vi "instrumentsInitialization.vi"(8 "error in":errorcluster, 11 "Instrument VISA in":T1={"AWG VISA"="AGTMY51400121", "Oscilloscope  VISA "="labosc4", "Integration Board IP"="172.16.7.43", "connection ID"=refnum, "report out"=refnum, "report file path"=path "C:/CTA/LevelTriggerBoardTest/TestsData/sumtrigger_delay/tmp"}) -> (0 "error out":errorcluster, 3 "Instrument VISA out":T1)   [LabVIEW 2012]
doc: "This VI initializes all the instrumentation needed to carry on several tests and also, establishes the communication with the Integration Board."
uses:
  <vilib>/Utility/NIReport.llb/NI_report.lvclass
  Sum_Abrilader/L0_Sum_Adder Folder/C/Program Files/National Instruments/LabVIEW 2012/instr.lib/Agilent 81150/Agilent 81150.lvlib
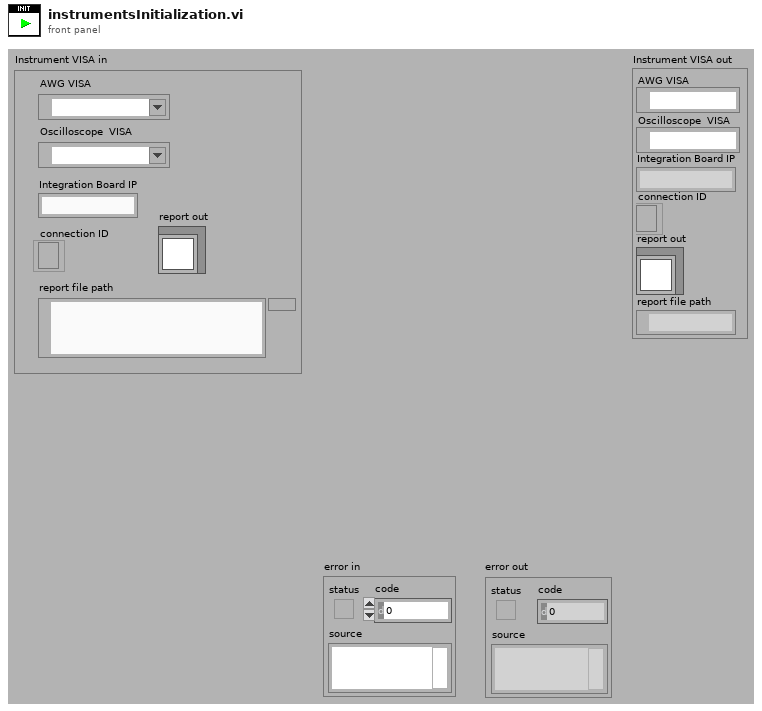
[diagram p1: front panel]
types:
  T1 = cluster{"AWG VISA":refnum<visa-resource-name>, "Oscilloscope  VISA ":refnum<visa-resource-name>, "Integration Board IP":string, "connection ID":refnum<k5>, "report out":refnum<class "NI_report.lvclass">, "report file path":path}
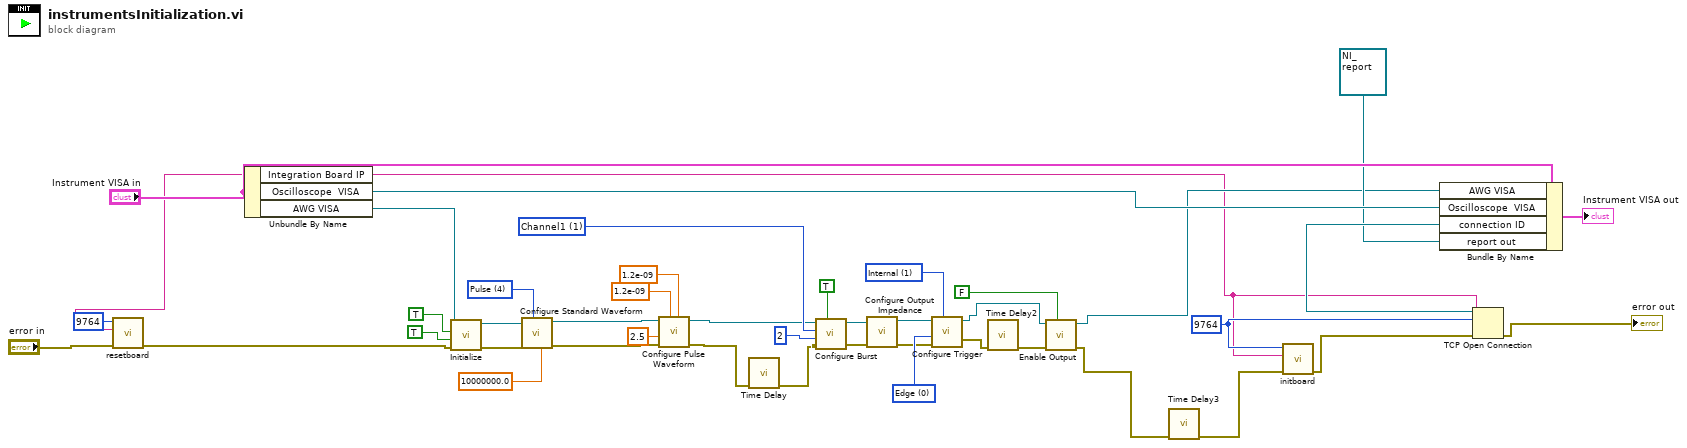
[diagram p0: block diagram]
diagram:
  w27 = u16 1 items=["Channel1"=1, "Channel2"=2] ("Channel (1: Channel1)")
  w34 = u16 4 items=["Sine", "Square", "Ramp Up", "Ramp Down", "Pulse", "Noise", "DC"] ("Waveform (0: Sine)")
  w6 = u16 9764 ("remote port or service name")
  w38 = u16 1 items=["Immediate", "Internal", "External", "Software Trigger Function"] ("Trigger Source (0: Immediate)")
  w43 = u16 0 items=["Edge", "Level"] ("Trigger Mode (0: Edge)")
  n1 = Unbundle By Name("Instrument VISA in") -> ("Integration Board IP"=w5:string, "Oscilloscope  VISA"=w23:refnum<visa-resource-name>, "AWG VISA"=w37:refnum<visa-resource-name>)
  n2 = call "resetboard.vi"("error in (no error)"="error in", "address"=w5, "remote port or service name"=u16 9764) -> ("error out"=w4:errorcluster)  [unwired: 7 in, 1 out]
  n3 = call <instrlib>:"Initialize.vi"("error in (no error)"=w4, "Reset (True)"=TRUE, "ID Query (True)"=TRUE, "VISA resource name"=w37) -> ("error out"=w32:errorcluster, "VISA resource name out"=w33:refnum<visa-resource-name>)  [unwired: 6 in]
  n4 = call <instrlib>:"Configure Standard Waveform.vi"("Frequency (1000.0 Hz)"=10000000.0, "Waveform (0: Sine)"=w34, "error in (no error)"=w32, "VISA resource name"=w33) -> ("error out"=w15:errorcluster, "VISA resource name out"=w13:refnum<visa-resource-name>)  [unwired: 6 in]
  n5 = call <instrlib>:"Configure Pulse Waveform.vi"("Trailing Edge Time (7.5E-9 Seconds)"=1.2e-09, "Leading Edge Time (7.5E-9 Seconds)"=1.2e-09, "error in (no error)"=w15, "Duty Cycle (50.0 %)"=2.5, "VISA resource name"=w13) -> ("error out"=w14:errorcluster, "VISA resource name out"=w12:refnum<visa-resource-name>)  [unwired: 5 in]
  n6 = call "Time Delay"("error in (no error)"=w14) -> ("error out"=w28:errorcluster)  [unwired: 10 in]
  n7 = call <instrlib>:"Configure Burst.vi"("Enable Burst (F: Disable)"=TRUE, "error in (no error)"=w28, "Burst Count (2)"=2, "Channel (1: Channel1)"=w27, "VISA resource name"=w12) -> ("error out"=w29:errorcluster, "VISA resource name out"=w30:refnum<visa-resource-name>)  [unwired: 5 in]
  n8 = call <instrlib>:"Configure Output Impedance.vi"("error in (no error)"=w29, "VISA resource name"=w30) -> ("error out"=w40:errorcluster, "VISA resource name out"=w39:refnum<visa-resource-name>)  [unwired: 8 in]
  n9 = call <instrlib>:"Configure Trigger.vi"("Trigger Source (0: Immediate)"=w38, "error in (no error)"=w40, "Trigger Mode (0: Edge)"=w43, "VISA resource name"=w39) -> ("error out"=w22:errorcluster, "VISA resource name out"=w18:refnum<visa-resource-name>)  [unwired: 6 in]
  n10 = call "Time Delay2"("error in (no error)"=w22) -> ("error out"=w19:errorcluster)  [unwired: 10 in]
  n11 = call <instrlib>:"Enable Output.vi"("Enable Output (T: Enable)"=FALSE, "error in (no error)"=w19, "VISA resource name"=w18) -> ("error out"=w3:errorcluster, "VISA resource name out"=w16:refnum<visa-resource-name>)  [unwired: 7 in]
  n12 = call "Time Delay3"("error in (no error)"=w3) -> ("error out"=w2:errorcluster)  [unwired: 10 in]
  n13 = call "initboard.vi"("error in (no error)"=w2, "address"=w5, "remote port or service name"=w6) -> ("error out"=w1:errorcluster)  [unwired: 8 in]
  n14 = TCP Open Connection(address=w5, remote port or service name=w6, error in (no error)=w1) -> (connection ID=w36:refnum<k5>, error out=→"error out":errorcluster)  [unwired: 2 in]
  n15 = Bundle By Name(cluster="Instrument VISA in", "AWG VISA"=w16, "Oscilloscope  VISA"=w23, "connection ID"=w36, "report out"=refnum<class "NI_report.lvclass"> refnum) -> (→"Instrument VISA out":T1)
